vi "PLC_LineOut.vi"(3 "error in (no error)":errorcluster, 4 "Selection":T1(ring), 5 "Resistor":i32, 6 "VISA resource name":refnum<visa-resource-name>) -> (0 "error out":errorcluster, 2 "VISA resource name out":refnum<visa-resource-name>)   [LabVIEW 2015]
panel:
  in  "PLC Address":u8
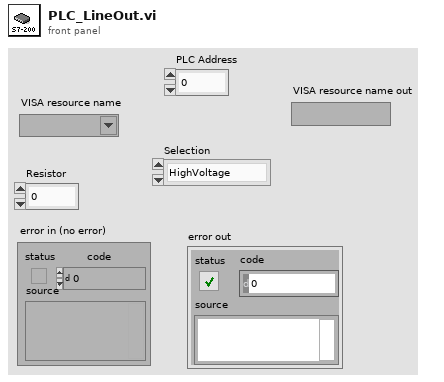
[diagram p1: front panel]
types:
  T1 = enum16{"HighVoltage", "LowVoltage", "Temperature", "AllOFF"}
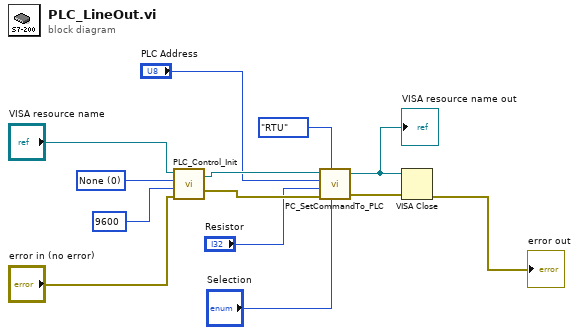
[diagram p0: block diagram]
diagram:
  w8 = u16 0 items=["None", "Odd", "Even", "Mark", "Space"] ("Parity")
  n1 = call "PLC_Control_Init.vi"("error in (no error)"="error in (no error)", "Baud Rate"=u32 9600, "Parity"=w8, "VISA resource name"="VISA resource name") -> ("error out"=w12:errorcluster, "VISA resource name out"=w11:refnum<visa-resource-name>)  [unwired: 2 in]
  n2 = call "PC_SetCommandTo_PLC.vi"("VISA resource name"=w11, "Mode"=enum16{"RTU", "ASCII"}."RTU", "PLC Address"="PLC Address", "Resistor"="Resistor", "Selection"="Selection", "error in (no error)"=w12) -> ("VISA resource name out"=w1:refnum<visa-resource-name>, "error out"=w13:errorcluster)  [unwired: 1 in]
  "VISA resource name out" <- w1
  n3 = VISA Close(VISA resource name=w1, error in (no error)=w13) -> (error out=→"error out":errorcluster)
